vi "putMirrorForceData.vi"(8 "error in (no error)":errorcluster, 10 "TelemetryMirrorForceData":T1, 11 "M1M3SAL in":refnum<class "M1M3SAL.lvclass">) -> (0 "error out":errorcluster, 3 "M1M3SAL out":refnum<class "M1M3SAL.lvclass">)   [LabVIEW 2016, in "M1M3SupportCommunicator.lvlib" / "M1M3SAL.lvclass"]
uses:
  M1M3SAL.lvclass
  DataTypes/Topics/TelemetryMirrorForceData.ctl
  DataTypes/Topics/Parts/Timestamp.ctl
  DataTypes/MessageHeader.ctl
  DataTypes/MessageTypes.ctl
  DataTypes/MessageTopics.ctl
  Common_RT_Utilities/U8ArrayBuilderAutoIndexing/U8ArrayBuilderAutoIndexing.lvclass
  M1M3SupportCommunicator.lvlib
  DataTypes/Topics/M1M3SupportTopics.lvlib
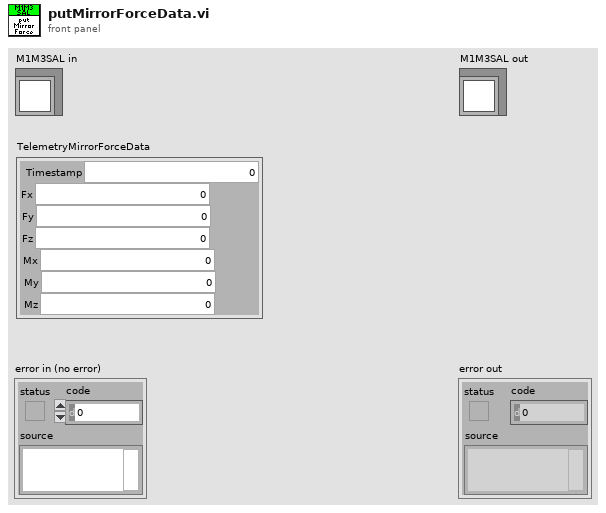
[diagram p1: front panel]
types:
  T1 = typedef "M1M3SupportTopics.lvlib/TelemetryMirrorForceData.ctl" = cluster{"Timestamp":T2, "Fx":dbl, "Fy":dbl, "Fz":dbl, "Mx":dbl, "My":dbl, "Mz":dbl}
  T2 = typedef "M1M3SupportTopics.lvlib/Timestamp.ctl" = dbl
  T3 = typedef "M1M3SupportCommunicator.lvlib/MessageHeader.ctl" = cluster{"Type":T4, "Topic":T5, "Size":i32}
  T4 = typedef "M1M3SupportCommunicator.lvlib/MessageTypes.ctl" = enum8{"None", "PutSample", "GetNextSample", "LogEvent", "GetEvent", "IssueCommand", "CommandId", "WaitForCompletion", "AcceptCommand", "AckCommand"}
  T5 = typedef "M1M3SupportCommunicator.lvlib/MessageTopics.ctl" = enum8{"None", "ForceActuatorData", "MirrorForceData", "HardpointData", "AirData", "DynamicData", "FPGAData", "IMSData", "ForceActuatorStatus", "ElevationData", "HardpointStatus", "HardpointActuatorChase", "AirStatus", "ForceActuatorSafetyChecks", "ForceActuatorTest", "ActuatorBroadcastCounter", "StatusChecks", "CellChecks", "HardpointActuatorBreakaway", "RaiseMirrorComplete", "ILCCommunication", "ElevationAngleChecks", "DetailedState", "ServoLoops", "ForceActuatorInfo", "LowerMirrorComplete", "HardpointActuatorInfo", "SettingsApplied", "ErrorCode", "StartupChecks", "SummaryState", "SettingVersions", "ActuatorTestStatus", "AppliedSettingsMatchStart", "Enable", "EnterMaintenance", "Standby", "AbortLowerM1M3", "ApplyAberrationByForces", "ApplyAOSCorrectionByBendingModes", "ClearAOSCorrection", "Start", "RaiseM1M3", "TestForceActuator", "LowerM1M3", "ApplyAOSCorrectionByForces", "Disable", "ApplyAberationByBendingMode", "TestHardpoint", "ManipulateM1M3", "ClearAberration", "Exit", "TestAir", "AbortRaiseM1M3", "MoveHardpointActuators", "ExitMaintenance", "Shutdown"}
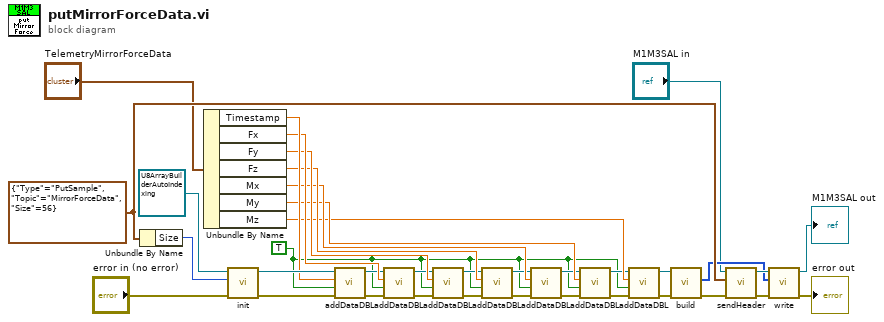
[diagram p0: block diagram]
diagram:
  w1 = TRUE ("OverrideSwapBytes")
  w35 = T3 {"Type"=enum."PutSample", "Topic"=enum."MirrorForceData", "Size"=56} ("MessageHeader")
  n1 = Unbundle By Name(w35) -> ("Size"=w34:i32)
  n2 = Unbundle By Name("TelemetryMirrorForceData") -> ("Timestamp"=w24:T2, "Fx"=w21:dbl, "Fy"=w20:dbl, "Fz"=w19:dbl, "Mx"=w18:dbl, "My"=w17:dbl, "Mz"=w16:dbl)
  n3 = call "init.vi"("error in (no error)"="error in (no error)", "Size"=w34, "U8ArrayBuilderAutoIndexing in"=refnum<class "U8ArrayBuilderAutoIndexing.lvclass"> refnum ("RTUtilities.lvlib:U8ArrayBuilderAutoIndexing.lvclass")) -> ("error out"=w23:errorcluster, "U8ArrayBuilderAutoIndexing out"=w25:refnum<class "U8ArrayBuilderAutoIndexing.lvclass">)  [unwired: 7 in]
  n4 = call "addDataDBL.vi"("error in (no error)"=w23, "OverrideSwapBytes"=w1, "Data"=w24, "U8ArrayBuilderAutoIndexing in"=w25) -> ("error out"=w8:errorcluster, "U8ArrayBuilderAutoIndexing out"=w15:refnum<class "U8ArrayBuilderAutoIndexing.lvclass">)  [unwired: 6 in]
  n5 = call "addDataDBL.vi"("error in (no error)"=w8, "OverrideSwapBytes"=w1, "Data"=w21, "U8ArrayBuilderAutoIndexing in"=w15) -> ("error out"=w7:errorcluster, "U8ArrayBuilderAutoIndexing out"=w14:refnum<class "U8ArrayBuilderAutoIndexing.lvclass">)  [unwired: 6 in]
  n6 = call "addDataDBL.vi"("error in (no error)"=w7, "OverrideSwapBytes"=w1, "Data"=w20, "U8ArrayBuilderAutoIndexing in"=w14) -> ("error out"=w6:errorcluster, "U8ArrayBuilderAutoIndexing out"=w13:refnum<class "U8ArrayBuilderAutoIndexing.lvclass">)  [unwired: 6 in]
  n7 = call "addDataDBL.vi"("error in (no error)"=w6, "OverrideSwapBytes"=w1, "Data"=w19, "U8ArrayBuilderAutoIndexing in"=w13) -> ("error out"=w5:errorcluster, "U8ArrayBuilderAutoIndexing out"=w12:refnum<class "U8ArrayBuilderAutoIndexing.lvclass">)  [unwired: 6 in]
  n8 = call "addDataDBL.vi"("error in (no error)"=w5, "OverrideSwapBytes"=w1, "Data"=w18, "U8ArrayBuilderAutoIndexing in"=w12) -> ("error out"=w4:errorcluster, "U8ArrayBuilderAutoIndexing out"=w11:refnum<class "U8ArrayBuilderAutoIndexing.lvclass">)  [unwired: 6 in]
  n9 = call "addDataDBL.vi"("error in (no error)"=w4, "OverrideSwapBytes"=w1, "Data"=w17, "U8ArrayBuilderAutoIndexing in"=w11) -> ("error out"=w3:errorcluster, "U8ArrayBuilderAutoIndexing out"=w10:refnum<class "U8ArrayBuilderAutoIndexing.lvclass">)  [unwired: 6 in]
  n10 = call "addDataDBL.vi"("error in (no error)"=w3, "OverrideSwapBytes"=w1, "Data"=w16, "U8ArrayBuilderAutoIndexing in"=w10) -> ("error out"=w2:errorcluster, "U8ArrayBuilderAutoIndexing out"=w9:refnum<class "U8ArrayBuilderAutoIndexing.lvclass">)  [unwired: 6 in]
  n11 = call "build.vi"("error in (no error)"=w2, "U8ArrayBuilderAutoIndexing in"=w9) -> ("error out"=w31:errorcluster, "Array"=w32:u8[])  [unwired: 7 in, 1 out]
  n12 = call "sendHeader.vi"("error in (no error)"=w31, "MessageHeader"=w35, "M1M3SAL in"="M1M3SAL in") -> ("error out"=w30:errorcluster, "M1M3SAL out"=w33:refnum<class "M1M3SAL.lvclass">)  [unwired: 7 in]
  n13 = call "write.vi"("error in (no error)"=w30, "Data"=w32, "M1M3SAL in"=w33) -> ("error out"=→"error out":errorcluster, "M1M3SAL out"=→"M1M3SAL out":refnum<class "M1M3SAL.lvclass">)  [unwired: 7 in]
